vi "Save Parameters 2 File (uSMC).vi"(3 "error in (no error)":errorcluster, 4 "SMIndex":i32, 5 "Path":path) -> (0 "error out":errorcluster)   [LabVIEW 2010, in "SignalWriterMH110203USBStepperMotor.lvclass"]
uses:
  SignalWriterMH110203USBStepperMotor.lvclass
  <vilib>/Utility/error.llb/DialogType.ctl
  class_data.vi
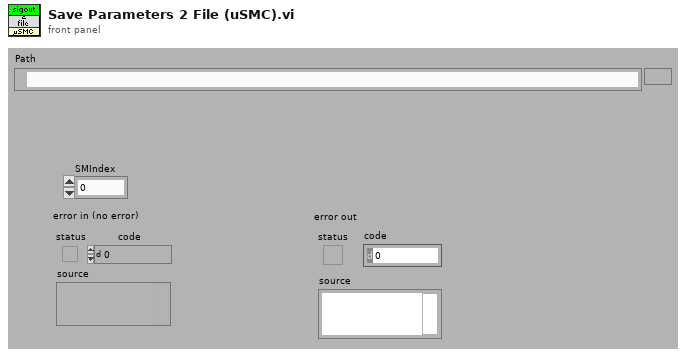
[diagram p1: front panel]
types:
  T1 = enum16{"open", "open or create", "create or replace", "create", "open (read only)"}
  T2 = typedef "SignalWriterMH110203USBStepperMotor.lvclass/Set Parameters (uSMC).ctl" = cluster{"Acceleration Time":u8, "Deceleration Time":u8, "Reduce Current Timeout":u16, "Buttons Timeout 1":u16, "Buttons Timeout 2":u16, "Buttons Timeout 3":u16, "Buttons Timeout 4":u16, "Buttons Timeout Reset":u16, "Buttons Timeout DblClick":u16, "Reset Speed":u16, "Buttons Speed 1":u16, "Buttons Speed 2":u16, "Buttons Speed 3":u16, "Buttons Speed 4":u16, "Max Backlash":u16, "Start Pos":i32, "RTdelta":u16, "RTMinError":u16, "Maximum Temperature":u16, "Sync Duration":u8, "Backlash Speed":u16, "EncVSCP":u8, "Steps Per Revolution":i32, "Encoder Pulses Per Rev-on":i32}
  T3 = typedef "SignalWriterMH110203USBStepperMotor.lvclass/GoTo Control (uSMC).ctl" = cluster{"Step motor ID":string, "SMname":string, "Backlash":u16, "wait for input sygnal to start":bool, "use slow start/stop":bool, "units name":string, "Maximum speed":dbl, "speed":dbl, "step":u8, "point 1 ticks":i32, "point 2 ticks":i32, "point 1 units":dbl, "point 2 units":dbl, "Limit Switch standoff":dbl, "Zero Value":dbl, "Destination Position":dbl, "force backlash":bool, "power off when stop":bool, "POff delay":dbl, "positioner name":string, "R, Ohm":dbl, "I, mA":dbl, "Positioner's Type":u16, "Reset Direction":bool, "Manufacturer":string, "Model":string, "Scheme":string, "FirmwareVer":string}
  T4 = cluster{"Cur Pos Units":dbl, "Set Cur Pos units":dbl, "Lo Limit Units":dbl, "Hi Limit Units":dbl, "Cur Pos Ticks":i32, "Set Cur Pos ticks":i32, "Lo Limit Ticks":i32, "Hi Limit Ticks":i32, "Minimal Value":dbl, "Maximal Value":dbl}[]
  T5 = typedef "SignalWriterMH110203USBStepperMotor.lvclass/Mode Control (uSMC).ctl" = cluster{"Turn Buttons Off":bool, "Reduce Current":bool, "Power Off and Make a Whole Step":bool, "Emergency Power Off":bool, "Limit Switch 1 True State":bool, "Limit Switch 2 True State":bool, "Rotary Transducer TRUE State":bool, "Swap Limit Switches":bool, "Limit Switch 1 Operation Enabled":bool, "Limit Switch 2 Operation Enabled":bool, "Rotary Transducer Operation Enabled":bool, "Rotary Transducer Operation Select":bool, "Button 1 True State":bool, "Button 2 True State":bool, "Swap Buttons":bool, "Reset Rotary Transducer Check Positions":bool, "Output Syncronization Enabled":bool, "Reset Output Sync Count":bool, "Sync Operation":bool, "Sync Count":u32, "Power":bool, "Invert Sync Polarity":bool, "Use Encoder":bool, "Invert Encoder Direction":bool, "Reset Encoder To 0":bool, "Reset SM Enc Pos to Enc Pos":bool}
  T6 = cluster{"Cur Pos Units":dbl, "Set Cur Pos units":dbl, "Lo Limit Units":dbl, "Hi Limit Units":dbl, "Cur Pos Ticks":i32, "Set Cur Pos ticks":i32, "Lo Limit Ticks":i32, "Hi Limit Ticks":i32, "Minimal Value":dbl, "Maximal Value":dbl}
  T7 = cluster{"Mode Defalults":T5, "Parameters Defalut":T2, "Position Default":cluster{"Cur Pos Units":dbl, "Set Cur Pos units":dbl, "Lo Limit Units":dbl, "Hi Limit Units":dbl, "Cur Pos Ticks":i32, "Set Cur Pos ticks":i32, "Lo Limit Ticks":i32, "Hi Limit Ticks":i32, "Minimal Value":dbl, "Maximal Value":dbl}, "StartPlus Default":T3}
  T8 = typedef "DialogType.ctl" = u16
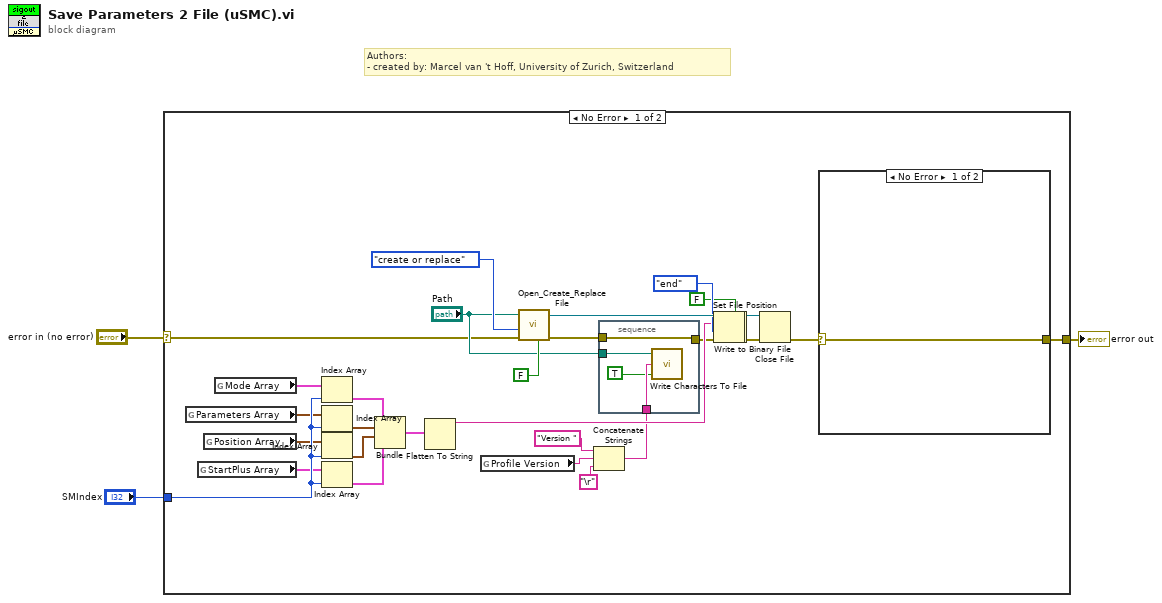
[diagram p0: block diagram]
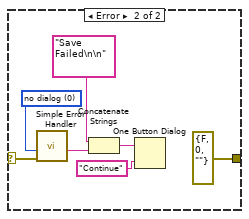
[diagram p2: hidden frame]
diagram:
  # "Authors: \n- created by: Marcel van 't Hoff, University of Zurich, Switzerland"
  n1 = case shown="No Error" "error in (no error)" {
    selector: "error in (no error)" -> [w4 w46]
    tunnel: "SMIndex" -> [w28 _]
    tunnel: [w21 w46] -> w2
    frame No Error {
      n2 = global read "class_data.vi" "Parameters Array"() -> (w10:T2[])
      n3 = global read "class_data.vi" "StartPlus Array"() -> (w8:T3[])
      n4 = global read "class_data.vi" "Position Array"() -> (w11:T4)
      n5 = global read "class_data.vi" "Mode Array"() -> (w9:T5[])
      n6 = Index Array(array=w9, index=w28) -> (element=w27:T5)
      n7 = Index Array(array=w10, index=w28) -> (element=w26:T2)
      n8 = Index Array(array=w11, index=w28) -> (element=w25:T6)
      n9 = Index Array(array=w8, index=w28) -> (element=w23:T3)
      n10 = Bundle("Mode Defalults"=w27, "Parameters Defalut"=w26, "Position Default"=w25, "StartPlus Default"=w23) -> (w24:T7)  [unwired: 1 in]
      n11 = Flatten To String(anything=w24) -> (data string=w29:string)  [unwired: 3 in, 2 out]
      n12 = global read "class_data.vi" "Profile Version"() -> (w12:string)
      n13 = call <vilib>:"Open_Create_Replace File.vi"("advisory dialog? (display:T)"=FALSE, "error in (no error)"=w4, "function (open:0)"=T1."create or replace", "file path"="Path") -> ("error out"=w14:errorcluster, "refnum"=w32:refnum<file>)  [unwired: 4 in, 2 out]
      n14 = Concatenate Strings("Version " ("string"), w12, "\r") -> (w16:string)
      n15 = stacked-sequence {
        tunnel: w16 -> [w37]
        tunnel: "Path" -> [w36]
        tunnel: w14 -> [w35]
        tunnel: [w35] -> w13
        frame #0 {
          n16 = call <vilib>:"Write Characters To File.vi"("append to file? (new file:F)"=TRUE, "character string"=w37, "file path (dialog if empty)"=w36) -> ()  [unwired: 2 in, 1 out]
        }
      }
      n17 = Set File Position(refnum=w32, from (0:start)=enum16{"start", "end", "current"}."end" ("pos mode (0:2)"), error in=w13) -> (refnum out=w7:refnum<file>, error out=w6:errorcluster)  [unwired: 1 in]
      n18 = Write to Binary File(file (use dialog)=w7, data=w29, error in=w6, 5:FALSE ("prepend array or string size? (T)")) -> (refnum out=w20:refnum<file>, error out=w19:errorcluster)  [unwired: 2 in, 1 out]
      n19 = Close File(refnum=w20, error in=w19) -> (error out=w22:errorcluster)  [unwired: 1 out]
      n20 = case shown="No Error" w22 {
        selector: w22 -> [w38 w44]
        tunnel: [w38 errorcluster {"status"=FALSE, "code"=0, "source"=""} ("error IO")] -> w21
        frame No Error {
        }
        frame Error {
          w43 = T8 0 items=["no dialog", "OK message", "continue or stop message", "OK message + warnings", "continue/stop + warnings"] ("type of dialog (OK msg:1)")
          n21 = call <vilib>:"Simple Error Handler.vi"("type of dialog (OK msg:1)"=w43, "error in (no error)"=w44) -> ("source out"=w42:string)  [unwired: 3 in, 4 out]
          n22 = Concatenate Strings("Save Failed\n\n" ("string"), w42) -> (w39:string)
          n23 = One Button Dialog(message=w39, button name ("OK")="Continue" ("T button name (\"OK\")")) -> ()  [unwired: 1 out]
        }
      }
    }
    frame Error {
    }
  }
  "error out" <- w2
